vi "TSL235R.vi"(0 "Irradiance µW/cm²":dbl) -> (1 "Output":dbl, 2 "Output Frequency (kHz)":dbl)   [LabVIEW 2013]
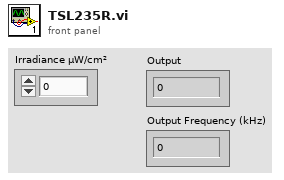
[diagram p1: front panel]
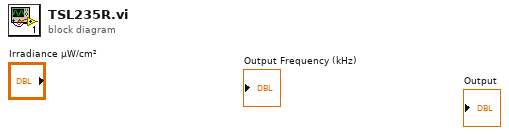
[diagram p0: block diagram]
diagram:
